vi "Read Transport.vi"(11 "Base Attributes in":refnum<class "Base Attributes.lvclass">) -> (2 "Transport":refnum<class "Transport.lvclass">)   [LabVIEW 2025, in "jettl.lvlib" / "Base Attributes.lvlib" / "Base Attributes.lvclass"]
uses:
  Base Attributes.lvclass
  Transport/Transport.lvclass
  Base Attributes.lvclass/Base Attributes.ctl
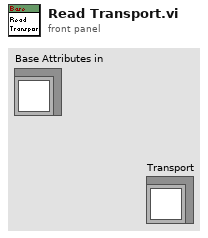
[diagram p1: front panel]
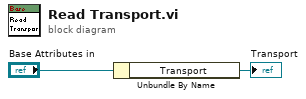
[diagram p0: block diagram]
diagram:
  n1 = Unbundle By Name("Base Attributes in") -> ("Transport"=→"Transport":refnum<class "Transport.lvclass">)
